vi "getLastWarning.vi"(8 "error in (no error)":errorcluster, 11 "VGS_RemoteControlClient in":refnum<class "VGS_RemoteControlClient.lvclass">) -> (0 "error out":errorcluster, 2 "LastWarning":string, 3 "VGS_RemoteControlClient out":refnum<class "VGS_RemoteControlClient.lvclass">)   [LabVIEW 2022 SP3, in "LV_VGS.lvlib" / "VGS_RemoteControlClient.lvclass"]
doc: "<B>Returns the last stored warning and resets the warning to NoWarning. </B>\n\nParameters\nhandle A valid remote handle. \n\nEmit error RemoteControlServiceIsNotAvailableException if the remote control service doesn't run. \nEmit error GenericRemoteControlErrorException if an internal error occurs. \nEmit error InvalidRemoteHandleException if the remote handle is not valid."
uses:
  VGS_RemoteControlClient.lvclass
  VGS_RemoteControlClient.lvclass/VGS_RemoteControlClient.ctl
  C:/Users/Andrey/Documents/GitHub/LV_VGS/vgs_project.dll
  vgs_project.dll
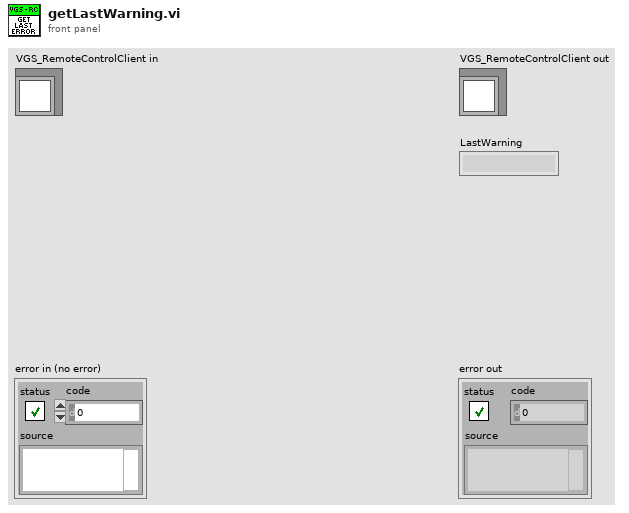
[diagram p1: front panel]
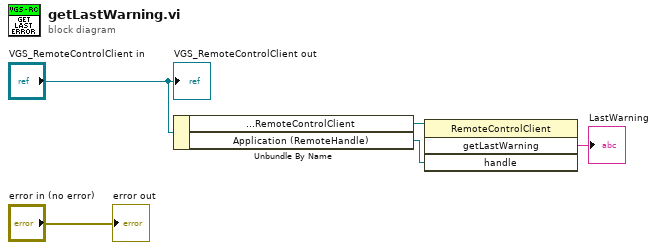
[diagram p0: block diagram]
diagram:
  n1 = Unbundle By Name("VGS_RemoteControlClient in") -> ("VGS.Project.Interop.RemoteControlClient"=w2:refnum<k24>, "Application (RemoteHandle)"=w1:refnum<k24>)
  n2 = invoke class="RemoteControlClient" method="getLastWarning"(reference=w2, "handle"=w1) -> ("getLastWarning"=→"LastWarning":string)  [unwired: 2 in, 3 out]
  "error out" <- "error in (no error)"
  "VGS_RemoteControlClient out" <- "VGS_RemoteControlClient in"
